vi "python code example.vi"() -> ()   [LabVIEW 2010]
panel:
  in  "exit":bool
  out "Notes":string="On the code, update this line with your file name.\n   FILENAME = 'MyCsvFileName.csv'\n\nThe data will be stored on the variable matrix.\n\nTo check the number of lines of the matrix, use:\n   print(len(matrix))"
  in  "Copy":bool
  in  "Python code to import the CSV file created":string="import csv, numpy\n\nFILENAME = 'MyCsvFileName.csv'\n\ndef convert(val): \n\ttry:\n\t\treturn float(val)\n\texcept:\n\t\treturn val\n\nwith open(FILENAME, 'r') as csvfile:\n\tspamreader = csv.reader(csvfile, delimiter=',', quotechar='|')\n\tvalues \t   = []\n\tmax_cols   = 0\n\tfor index, row in enumerate(spamreader):\n\t\tif index==0: continue\n\t\trow = list(map(convert, row))\n\t\tif len(row)>max_cols: max_cols=len(row)\n\t\tvalues.append(row)\n\n\tmatrix = []\n\tfor row in values:\n\t\trow = row + [None for x in range(max_cols-len(row))]\n\t\tmatrix.append(row)\n\n\tmatrix = numpy.array(matrix)"
  # "Python code to import the CSV file created"
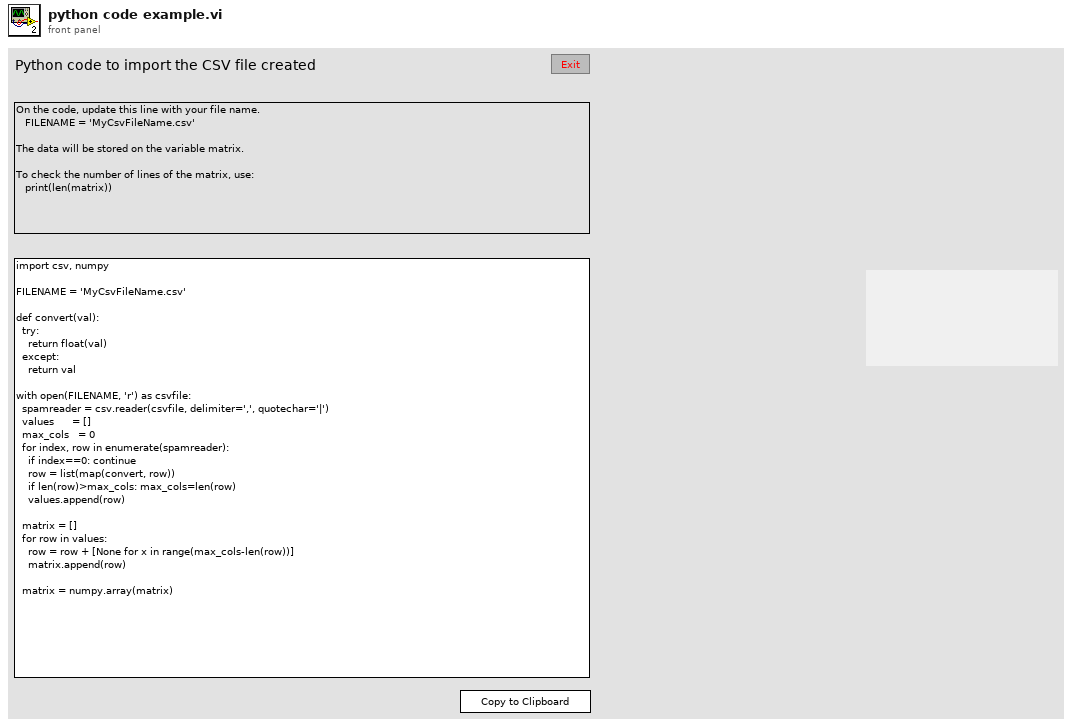
[diagram p1: front panel]
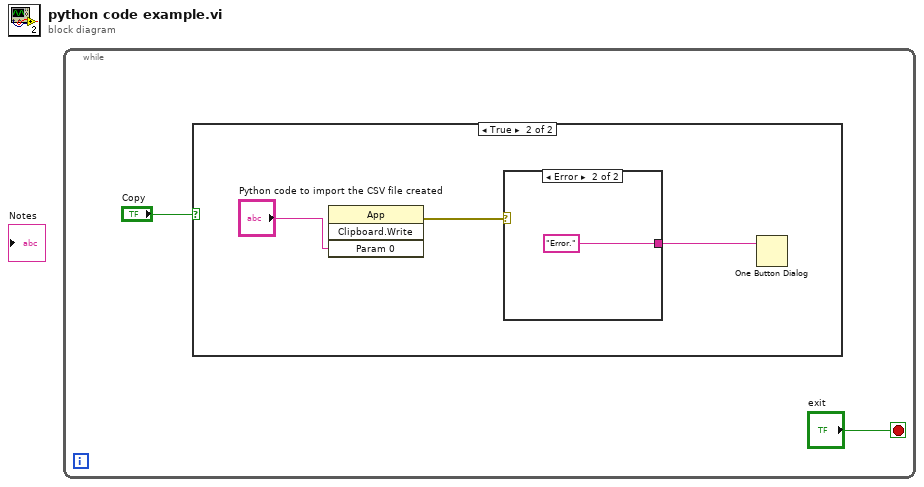
[diagram p0: block diagram]
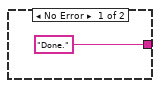
[diagram p3: hidden frame]
diagram:
  n1 = while {
    stop <- "exit" stop-if-true
    n2 = case shown="True" "Copy" {
      frame False {
      }
      frame True {
        n3 = invoke class="App" method="Clipboard.Write"("Param 0"="Python code to import the CSV file created") -> (error out=w4:errorcluster)  [unwired: 3 in, 3 out]
        n4 = case shown="Error" w4 {
          tunnel: ["Done." ("message") "Error." ("message")] -> w3
          frame No Error {
          }
          frame Error {
          }
        }
        n5 = One Button Dialog(message=w3) -> ()  [unwired: 1 in, 1 out]
      }
    }
  }
